vi "Save Config File.vi"(8 "error in (no error)":errorcluster, 10 "file path":path, 11 "DSF Configuration Reference in":T1) -> (0 "error out":errorcluster, 2 "file path out":path, 3 "DSF Configuration Reference out":T1)   [LabVIEW 2017, in "DSF Core.lvlib" / "Configuration Session.lvclass"]
uses:
  Configuration Session.lvclass
  DSF Config Data Ref.ctl
  DSF Config Data.ctl
  Internal DSF Configuration.ctl
  Typedefs/DSF Version Info.ctl
  Internal DSF Plugin with ID.ctl
  Internal DSF Plugin Info.ctl
  Typedefs/DSF Timing Info.ctl
  Typedefs/DSF Engine Plugin Thread Configuration.ctl
  Typedefs/DSF Settings Info.ctl
  Internal DSF Group with ID.ctl
  Internal DSF Group Info.ctl
  Internal DSF Transfer with ID.ctl
  Internal DSF Transfer Info.ctl
  Internal DSF Channel with ID.ctl
  Internal DSF Channel Info.ctl
  Internal DSF Settings with ID.ctl
  Internal DSF Settings Info.ctl
  DSF Core.lvlib
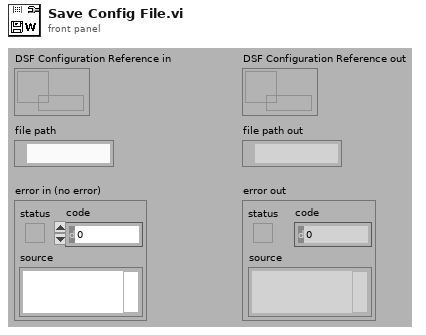
[diagram p1: front panel]
types:
  T1 = typedef "DSF Core.lvlib/Configuration Session.lvclass/DSF Config Data Ref.ctl" = refnum<data-value>
  T2 = enum16{"open", "replace", "create", "open or create", "replace or create", "replace or create with confirmation"}
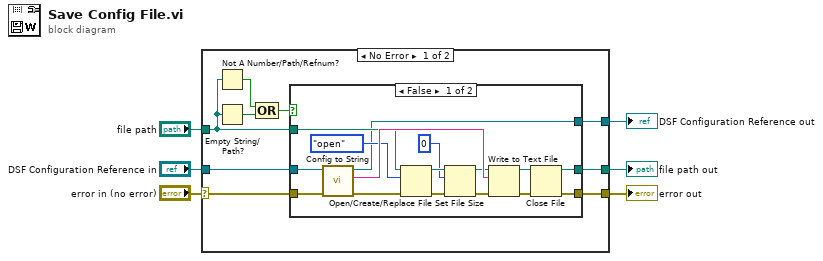
[diagram p0: block diagram]
diagram:
  n1 = case shown="No Error" "error in (no error)" {
    selector: "error in (no error)" -> [w8 w37]
    tunnel: [w15 w37] -> w5
    tunnel: [w14 w36] -> w3
    tunnel: "DSF Configuration Reference in" -> [w9 w36]
    tunnel: "file path" -> [w10 w35]
    tunnel: [w7 w35] -> w1
    frame No Error {
      n2 = Not A Number/Path/Refnum? ("Not A Number/Path/dsf refnum?")(number/path/refnum=w10) -> (NaN/Path/Refnum?=w13:bool)
      n3 = Empty String/Path?(string/path=w10) -> (empty?=w12:bool)
      n4 = Compound Arithmetic op=OR(w13, w12) -> (w11:bool)
      n5 = case shown="False" w11 {
        tunnel: [w29 w34] -> w15
        tunnel: w8 -> [w25 w34]
        tunnel: w10 -> [w26 w32]
        tunnel: w9 -> [w27 w33]
        tunnel: [w22 w33] -> w14
        tunnel: [w21 w32] -> w7
        frame False {
          n6 = call "Config to String.vi"("error in (no error)"=w25, "DSF Configuration Reference in"=w27) -> ("error out"=w24:errorcluster, "String"=w28:string, "DSF Configuration Reference out"=w22:T1)  [unwired: 7 out]
          n7 = Open/Create/Replace File(file path (use dialog)=w26, error in=w24, operation (0:open)=T2."open") -> (refnum out=w18:refnum<file>, error out=w20:errorcluster)  [unwired: 4 out]
          n8 = Set File Size(4:w20, 6:i64 0 ("size (in bytes)"), 7:w18) -> (0:w19:errorcluster, 3:w17:refnum<file>)
          n9 = Write to Text File(file (use dialog)=w17, text=w28, error in=w19) -> (refnum out=w31:refnum<file>, error out=w30:errorcluster)  [unwired: 2 out]
          n10 = Close File(refnum=w31, error in=w30) -> (path=w21:path, error out=w29:errorcluster)
        }
        frame True {
        }
      }
    }
    frame Error {
    }
  }
  "error out" <- w5
  "DSF Configuration Reference out" <- w3
  "file path out" <- w1
